vi "DetectTriggerGivenTrack.vi"(8 "error in (no error)":errorcluster, 9 "CameraFrame":i32, 10 "Track":T1, 11 "StimOnHeadBends in":refnum<class "StimOnHeadBends.lvclass">) -> (0 "error out":errorcluster, 2 "Triggered?":bool, 3 "StimOnHeadBends out":refnum<class "StimOnHeadBends.lvclass">)   [LabVIEW 2019, in "StimOnHeadBends.lvclass"]
uses:
  StimOnHeadBends.lvclass
  WormTrackCluster.ctl
  StimulusObject.lvclass
  TrackTerminationReasonEnum.ctl
  StimOnHeadBends.lvclass/StimOnHeadBends.ctl
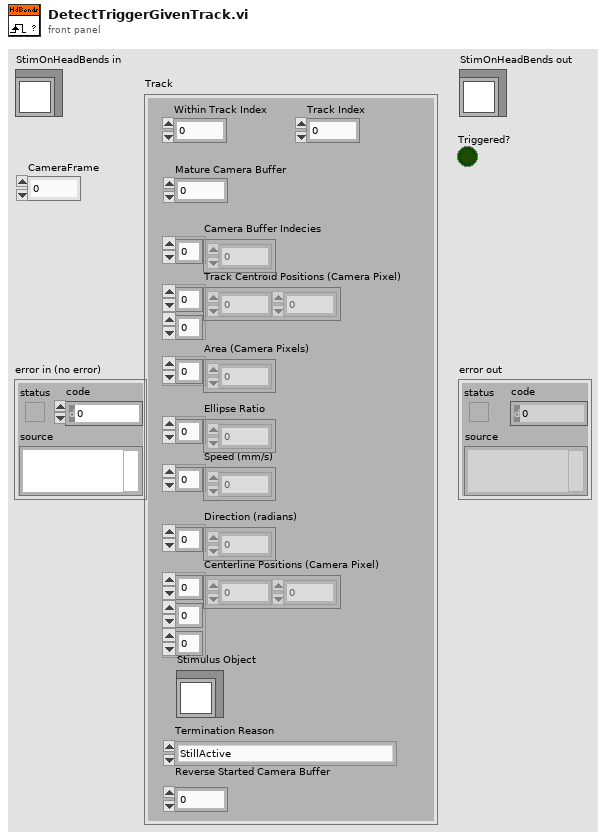
[diagram p1: front panel]
types:
  T1 = typedef "WormTrackCluster.ctl" = cluster{"Track Centroid Positions (Camera Pixel)":sgl[][], "Within Track Index":i32, "Camera Buffer Indecies":i32[], "Area (Camera Pixels)":i32[], "Speed (mm/s)":sgl[], "Direction (radians)":sgl[], "Centerline Positions (Camera Pixel)":sgl[][][], "Ellipse Ratio":sgl[], "Stimulus Object":refnum<class "StimulusObject.lvclass">, "Termination Reason":T2, "Track Index":i32, "Mature Camera Buffer":i32, "Reverse Started Camera Buffer":i32}
  T2 = typedef "TrackTerminationReasonEnum.ctl" = enum16{"StillActive", "MaxDisplacement", "NoBlobsLeft", "AreaIncrease", "AreaDecrease", "ExperimentEnded"}
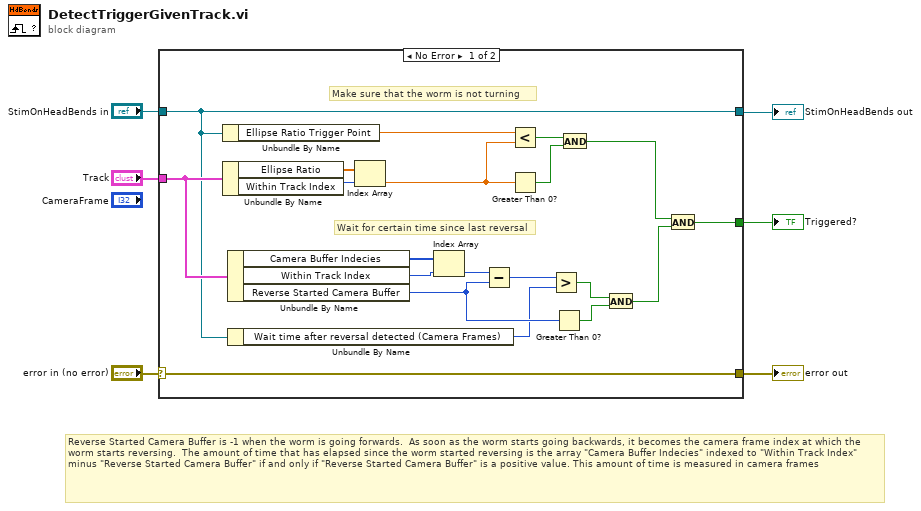
[diagram p0: block diagram]
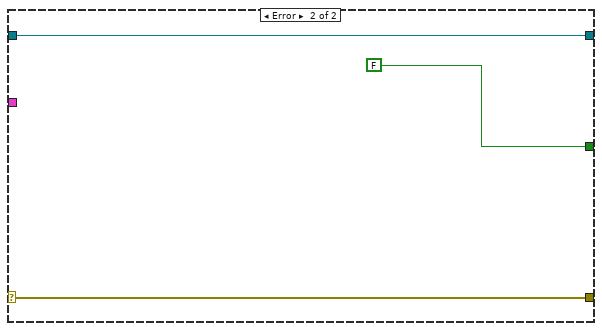
[diagram p2: hidden frame]
diagram:
  # "Reverse Started Camera Buffer is -1 when the worm is going forwards.  As soon as the worm starts going backwards, it becomes the camera frame index at which the worm starts reversing.  The amount of time that has elapsed since the worm started reversing is the array \"Camera Buffer Indecies\" indexed to \"Within Track Index\" minus \"Reverse Started Camera Buffer\" if and only if \"Reverse Started Camera Buffer\" is a positive value. This amount of time is measured in camera frames"
  n1 = case shown="No Error" "error in (no error)" {
    selector: "error in (no error)" -> [w26 w29]
    tunnel: [w26 w29] -> w1
    tunnel: "StimOnHeadBends in" -> [w10 w28]
    tunnel: [w10 w28] -> w3
    tunnel: "Track" -> [w11 _]
    tunnel: [w7 FALSE] -> w2
    frame No Error {
      # "Wait for certain time since last reversal"
      # "Make sure that the worm is not turning"
      n2 = Unbundle By Name(w10) -> ("Ellipse Ratio Trigger Point"=w23:sgl)
      n3 = Unbundle By Name(w11) -> ("Ellipse Ratio"=w25:sgl[], "Within Track Index"=w24:i32)
      n4 = Unbundle By Name(w11) -> ("Camera Buffer Indecies"=w19:i32[], "Within Track Index"=w18:i32, "Reverse Started Camera Buffer"=w15:i32)
      n5 = Unbundle By Name(w10) -> ("Wait time after reversal detected (Camera Frames)"=w12:i32)
      n6 = Index Array(array=w25, index=w24) -> (element=w20:sgl)
      n7 = Index Array(array=w19, index=w18) -> (element=w17:i32)
      n8 = Subtract(x=w17, y=w15) -> (x-y=w16:i32)
      n9 = Less?(x=w23, y=w20) -> (x < y?=w22:bool)
      n10 = Greater Than 0?(x=w20) -> (x > 0?=w21:bool)
      n11 = Greater?(x=w16, y=w12) -> (0:w14:bool)
      n12 = Greater Than 0?(x=w15) -> (x > 0?=w13:bool)
      n13 = And(x=w22, y=w21) -> (x .and. y?=w8:bool)
      n14 = And(x=w14, y=w13) -> (x .and. y?=w9:bool)
      n15 = And(x=w8, y=w9) -> (x .and. y?=w7:bool)
    }
    frame Error {
    }
  }
  "error out" <- w1
  "StimOnHeadBends out" <- w3
  "Triggered?" <- w2
